vi "Module Loop.vi"(8 "error in (no error)":errorcluster, 11 "System Status Module in":refnum<class "System Status Module.lvclass">) -> (0 "error out":errorcluster, 3 "System Status Module out":refnum<class "System Status Module.lvclass">)   [LabVIEW 2020, in "VolatusGUI.lvlib" / "System Status Module.lvclass"]
uses:
  System Status Module.lvclass
  C:/dev/lv20CE/relink/lv-volatus/Volatus/Module/Module.lvclass
  Client Row.ctl
  Volatus/Module/Module.lvclass/Module.ctl
  Volatus/MessageQ/MessageQ.lvclass/MessageQ.ctl
  System Status Module.lvclass/System Status Module.ctl
  Volatus/Module/Module.lvclass
  Config Updater Identity/Config Updater Identity.lvclass
  C:/dev/lv20CE/relink/lv-volatus/Volatus/Identity/Identity.lvclass
  <vilib>/Utility/error.llb/Error Cluster From Error Code.vi
  Volatus/MessageQ/MessageQ.lvclass
  GUI Helper/GUI Helper.lvclass
  Volatus/VolatusAPI/VolatusAPI.lvclass
  Volatus/Volatus.lvlib
panel:
  in  "Reload Config":bool
  in  "Manage Config":bool
  in  "Clients":T1[](array[typedef])
  # "Node"
  # "Alias"
  # "IP"
  # "App Ver"
  # "Cfg Ver"
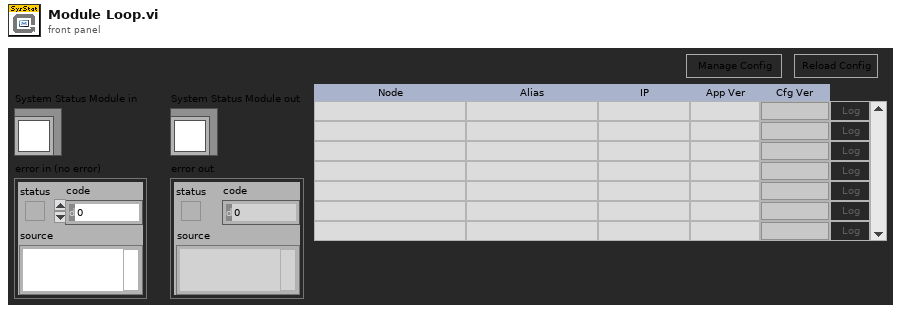
[diagram p1: front panel]
types:
  T1 = typedef "VolatusGUI.lvlib/System Status Module.lvclass/Client Row.ctl" = cluster{"Node":string, "Alias":string, "IP":string, "App Version":string, "Cfg Version":string, "Debug Log":bool, "Cfg Color":u32}
  T2 = enum32{"Invalid", "Standard", "Closed", "Hidden", "Minimized", "Maximized"}
  T3 = cluster{"Node":bool, "Alias":bool, "IP":bool, "App Version":bool, "Cfg Version":bool, "Debug Log":bool, "Cfg Color":bool}[]
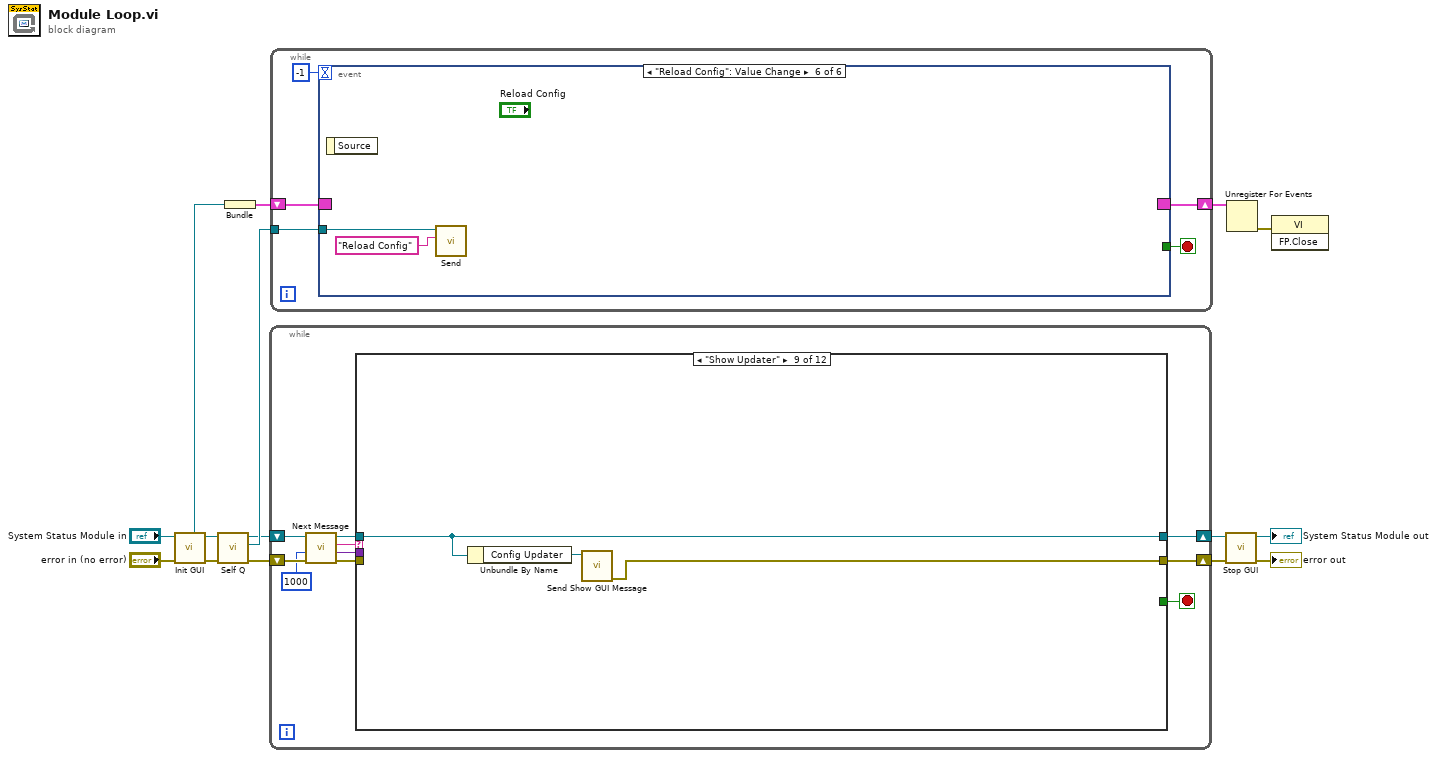
[diagram p0: block diagram]
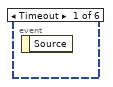
[diagram p2: hidden frame]
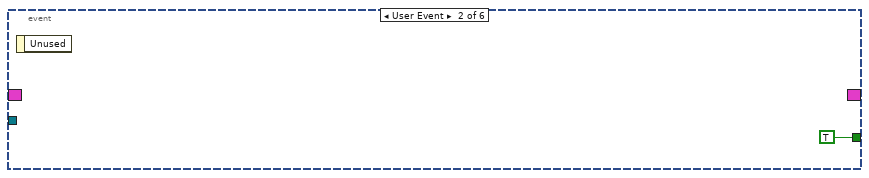
[diagram p3: hidden frame]
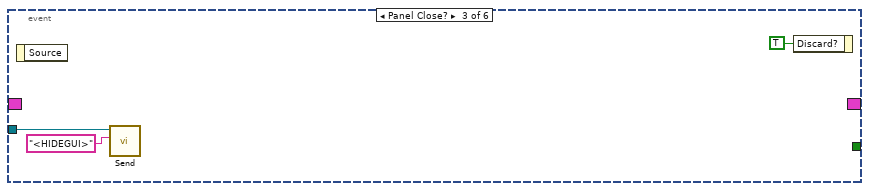
[diagram p4: hidden frame]
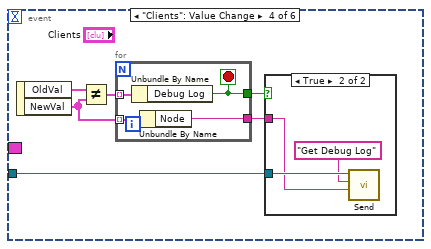
[diagram p5: hidden frame]
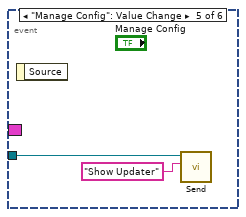
[diagram p7: hidden frame]
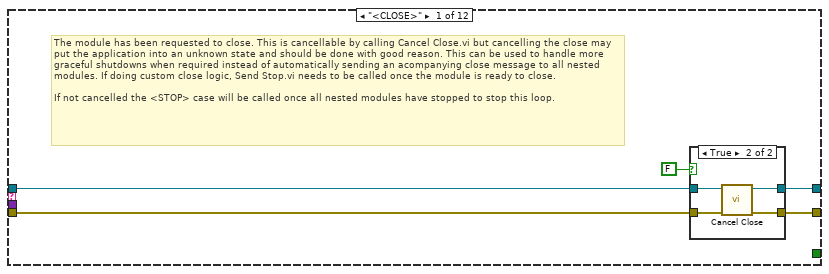
[diagram p8: hidden frame]
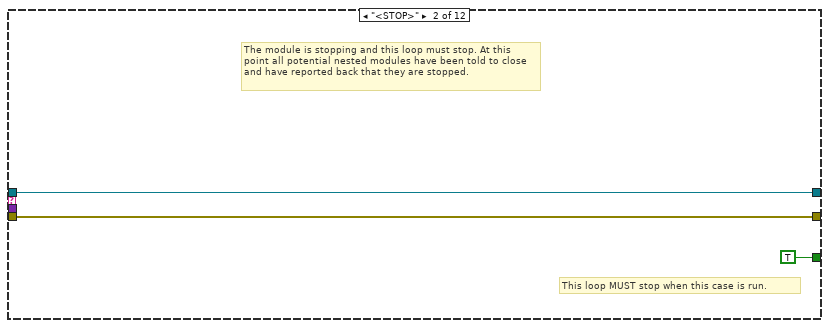
[diagram p10: hidden frame]
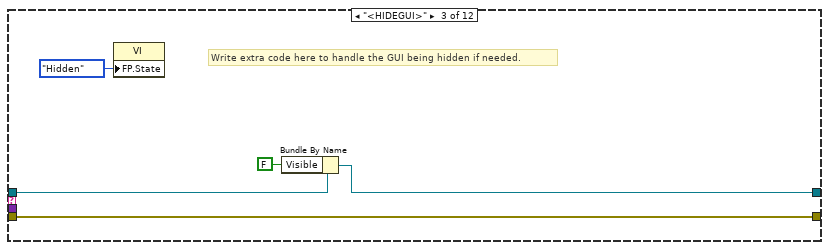
[diagram p11: hidden frame]
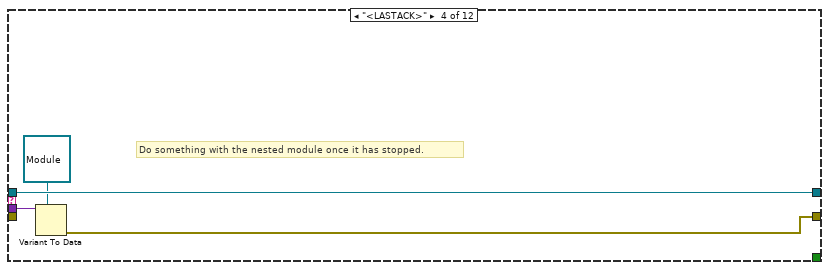
[diagram p12: hidden frame]
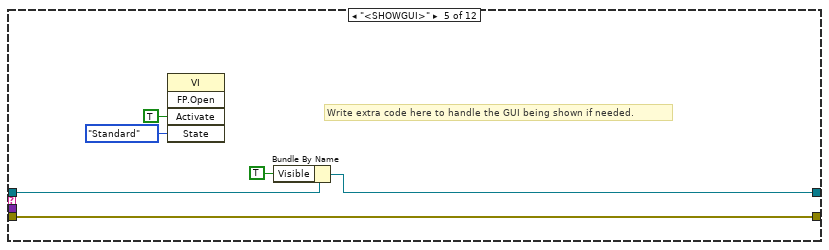
[diagram p13: hidden frame]
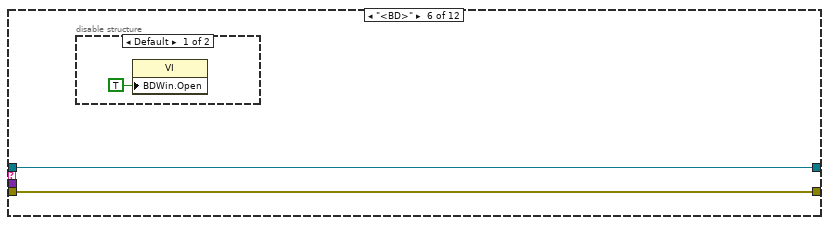
[diagram p14: hidden frame]
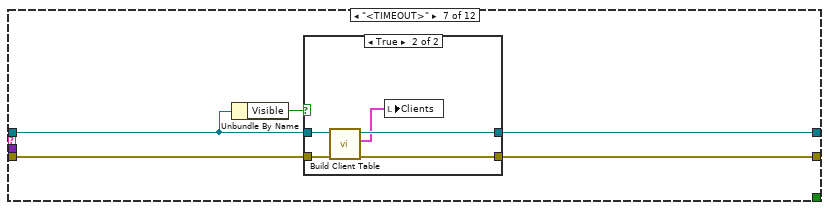
[diagram p16: hidden frame]
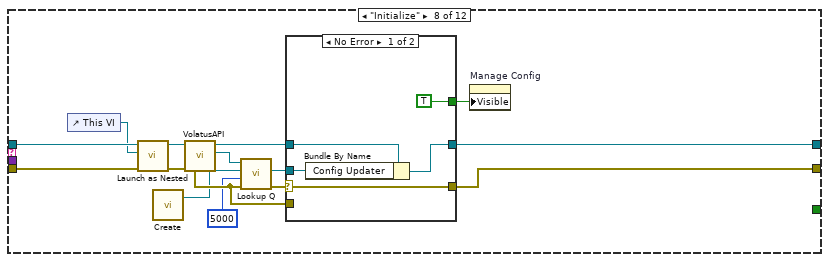
[diagram p18: hidden frame]
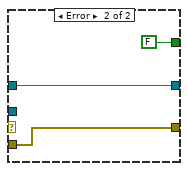
[diagram p19: hidden frame]
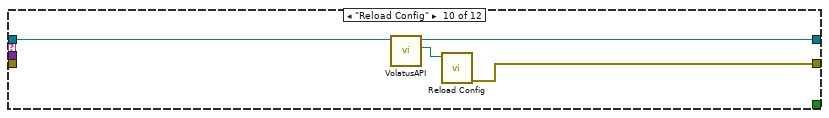
[diagram p20: hidden frame]
diagram:
  n1 = call "Init GUI.vi"("Module in"="System Status Module in") -> ("Module out"=w7:refnum<class "System Status Module.lvclass">, "Event Reg"=w12:refnum<event-registration>)  [unwired: 9 in]
  n2 = call "Self Q.vi"("Module in"=w7) -> ("Self Q"=w6:refnum<class "MessageQ.lvclass">, "Module out"=w5:refnum<class "System Status Module.lvclass">)  [unwired: 9 in]
  n3 = Bundle("Event Reg"=w12) -> (w8:cluster{"Event Reg":refnum<event-registration>})  [unwired: 1 in]
  n4 = while {
    shift-right: [w18] -> w10
    shift-left: w5 -> [w23]
    shift-right: [w17] -> w11
    shift-left: "error in (no error)" -> [w22]
    stop <- w16 stop-if-true
    n5 = call "Next Message.vi"("error in (no error)"=w22, "Timeout ms (-1)"=1000, "Module in"=w23) -> ("error out"=w21:errorcluster, "Data"=w15:variant, "ID"=w20:string, "Module out"=w19:refnum<class "System Status Module.lvclass">)  [unwired: 5 in]
    n6 = case shown="\"Show Updater\"" w20 {
      tunnel: w21 -> [w26 w36 w41 _ w51 w53 w60 w80 _ _ _ w107]
      tunnel: w19 -> [w27 w37 w42 w46 w52 w54 w57 w79 w92 w96 w103 w105]
      tunnel: [w25 w37 w39 w46 w48 w54 w58 w72 w92 w95 w100 w104] -> w18
      tunnel: [w24 w36 w41 w43 w51 w53 w59 w69 w90 w93 w97 w106] -> w17
      tunnel: [_ TRUE _ _ _ _ _ _ _ _ _ _] -> w16
      tunnel: w15 -> [_ _ _ w45 _ _ _ _ _ _ w102 _]
      frame "<CLOSE>" {
        # "The module has been requested to close. This is cancellable by calling Cancel Close.vi but cancelling the close may put the application into an unknown state and should be done with good reason. This can be used to handle more graceful shutdowns when required instead of automatically sending an acompanying close message to all nested modules. If doing custom close logic, Send Stop.vi needs to be called once the module is ready to close.\n\nIf not cancelled the <STOP> case will be called once all nested modules have stopped to stop this loop."
        n7 = case shown="True" FALSE {
          tunnel: w26 -> [w29 w34]
          tunnel: [w29 w33] -> w24
          tunnel: w27 -> [w30 w32]
          tunnel: [w30 w31] -> w25
          frame False {
          }
          frame True {
            n8 = call "Cancel Close.vi"("error in (no error)"=w34, "Module in"=w32) -> ("error out"=w33:errorcluster, "Module out"=w31:refnum<class "System Status Module.lvclass">)  [unwired: 8 in]
          }
        }
      }
      frame "<STOP>" {
        # "This loop MUST stop when this case is run."
        # "The module is stopping and this loop must stop. At this point all potential nested modules have been told to close and have reported back that they are stopped."
      }
      frame "<HIDEGUI>" {
        # "Write extra code here to handle the GUI being hidden if needed."
        n9 = property class="VI"("FP.State"=T2."Hidden" ("Front Panel Window:State")) -> ()  [unwired: 2 in, 2 out]
        n10 = Bundle By Name(cluster=w42, "Visible"=FALSE) -> (w39:refnum<class "System Status Module.lvclass">)
      }
      frame "<LASTACK>" {
        # "Do something with the nested module once it has stopped."
        n11 = Variant To Data(type=refnum<class "Module.lvclass"> refnum ("Volatus:Module"), Variant=w45) -> (error out=w43:errorcluster)  [unwired: 1 in, 1 out]
      }
      frame "<SHOWGUI>" {
        # "Write extra code here to handle the GUI being shown if needed."
        n12 = invoke class="VI" method="FP.Open"("Activate"=TRUE ("Activate?"), "State"=T2."Standard") -> ()  [unwired: 3 in, 5 out]
        n13 = Bundle By Name(cluster=w52, "Visible"=TRUE) -> (w48:refnum<class "System Status Module.lvclass">)
      }
      frame "<BD>" {
        n14 = disable-structure shown="Default" {
          frame condition #0 (active) {
            n15 = property class="VI"("BDWin.Open"=TRUE ("Block Diagram Window:Open")) -> ()  [unwired: 2 in, 2 out]
          }
          frame condition #1 {
          }
        }
      }
      frame "<TIMEOUT>" {
        n16 = Unbundle By Name(w57) -> ("Visible"=w56:bool)
        n17 = case shown="True" w56 {
          tunnel: w60 -> [w61 w67]
          tunnel: [w61 w66] -> w59
          tunnel: [w62 w65] -> w58
          tunnel: w57 -> [w62 w64]
          frame False {
          }
          frame True {
            n18 = call "Build Client Table.vi"("error in (no error)"=w67, "System Status Module in"=w64) -> ("error out"=w66:errorcluster, "Clients"=w63:T1[], "System Status Module out"=w65:refnum<class "System Status Module.lvclass">)  [unwired: 7 in]
            n19 = local write "Clients"(w63) -> ()
          }
        }
      }
      frame "Initialize" {
        n20 = control-ref of="This VI"() -> (w77:refnum<vi>)
        n21 = call "Launch as Nested.vi"("error in (no error)"=w80, "GUI"=w77, "Parent in"=w79) -> ("error out"=w81:errorcluster, "Parent"=w78:refnum<class "System Status Module.lvclass">)  [unwired: 6 in, 1 out]
        n22 = call "Create.vi"() -> ("Config Updater Identity"=w73:refnum<class "Config Updater Identity.lvclass">)  [unwired: 7 in]
        n23 = call "VolatusAPI.vi"("Module in"=w78) -> ("VolatusAPI"=w75:refnum<class "VolatusAPI.lvclass">, "Module out"=w76:refnum<class "System Status Module.lvclass">)  [unwired: 9 in]
        n24 = call "Lookup Q.vi"("error in (no error)"=w81, "Timeout ms (0)"=5000, "Identity"=w73, "VolatusAPI in"=w75) -> ("error out"=w70:errorcluster, "MessageQ"=w71:refnum<class "MessageQ.lvclass">)  [unwired: 5 in, 1 out]
        n25 = case shown="No Error" w70 {
          selector: w70 -> [w83 _]
          tunnel: w76 -> [w86 w88]
          tunnel: [w85 w88] -> w72
          tunnel: w71 -> [w84 _]
          tunnel: [w83 w89] -> w69
          tunnel: w81 -> [_ w89]
          tunnel: [TRUE FALSE] -> w68
          frame No Error {
            n26 = Bundle By Name(cluster=w86, "Config Updater"=w84) -> (w85:refnum<class "System Status Module.lvclass">)
          }
          frame Error {
          }
        }
        n27 = property on="Manage Config" class="Bool"("Visible"=w68) -> ()  [unwired: 2 in, 2 out]
      }
      frame "Show Updater" {
        n28 = Unbundle By Name(w92) -> ("Config Updater"=w91:refnum<class "MessageQ.lvclass">)
        n29 = call "Send Show GUI Message.vi"("MessageQ"=w91) -> ("error out"=w90:errorcluster)  [unwired: 10 in]
      }
      frame "Reload Config" {
        n30 = call "VolatusAPI.vi"("Module in"=w96) -> ("VolatusAPI"=w94:refnum<class "VolatusAPI.lvclass">, "Module out"=w95:refnum<class "System Status Module.lvclass">)  [unwired: 9 in]
        n31 = call "Reload Config.vi"("VolatusAPI in"=w94) -> ("error out"=w93:errorcluster)  [unwired: 9 in, 1 out]
      }
      frame "Get Debug Log" {
        n32 = Variant To Data(type="", Variant=w102) -> (data=w99:string, error out=w98:errorcluster)  [unwired: 1 in]
        n33 = call "Get Debug Log.vi"("error in (no error)"=w98, "Node"=w99, "System Status Module in"=w103) -> ("error out"=w97:errorcluster, "System Status Module out"=w100:refnum<class "System Status Module.lvclass">)  [unwired: 7 in]
      }
      frame Default {
        n34 = call "Report Unhandled Message ID.vi"("error in (no error)"=w107, "Module in"=w105) -> ("error out"=w106:errorcluster, "Module out"=w104:refnum<class "System Status Module.lvclass">)  [unwired: 8 in]
      }
    }
  }
  n35 = while {
    tunnel: w6 -> [w112]
    shift-right: [w110] -> w9
    shift-left: w8 -> [w111]
    stop <- w109 stop-if-true
    n36 = event shown="[5] \"Reload Config\": Value Change" {
      selector: w111 -> [_ _ _ _ _ _]
      dyn-events: [_ _ _ _ _ _] -> w110
      timeout: -1 -> [_ _ _ _ _ _]
      tunnel: w112 -> [_ _ w115 w117 w131 w133]
      tunnel: [_ TRUE _ _ _ _] -> w109
      event Timeout {
        n37 = event-data() -> ()  [unwired: 1 in, 1 out]
      }
      event User Event {
        n38 = event-data() -> ()  [unwired: 1 in, 1 out]
      }
      event Panel Close? {
        n39 = event-data() -> ()  [unwired: 1 in, 1 out]
        n40 = call "Send.vi"("ID"="<HIDEGUI>", "MessageQ in"=w115) -> ()  [unwired: 8 in, 2 out]
        n41 = event-data("Discard?"=TRUE) -> ()  [unwired: 1 in, 1 out]
      }
      event "Clients": Value Change {
        n42 = event-data() -> ("OldVal"=w122:T1[], "NewVal"=w120:T1[])  [unwired: 1 in]
        n43 = Not Equal?(x=w122, y=w120) -> (x != y?=w121:T3)
        n44 = for {
          tunnel: w121 -> [w129] mode=indexing
          tunnel: w120 -> [w128] mode=indexing
          tunnel: [w127] -> w118
          tunnel: [w126] -> w119
          stop <- w126 stop-if-true
          n45 = Unbundle By Name(w129) -> ("Debug Log"=w126:bool)
          n46 = Unbundle By Name(w128) -> ("Node"=w127:string)
        }
        n47 = case shown="True" w119 {
          tunnel: w118 -> [_ w123]
          tunnel: w117 -> [_ w125]
          frame False {
          }
          frame True {
            n48 = call "Send.vi"("Data"=w123, "ID"="Get Debug Log", "MessageQ in"=w125) -> ()  [unwired: 7 in, 2 out]
          }
        }
      }
      event "Manage Config": Value Change {
        n49 = event-data() -> ()  [unwired: 1 in, 1 out]
        n50 = call "Send.vi"("ID"="Show Updater", "MessageQ in"=w131) -> ()  [unwired: 8 in, 2 out]
      }
      event "Reload Config": Value Change {
        n51 = event-data() -> ()  [unwired: 1 in, 1 out]
        n52 = call "Send.vi"("ID"="Reload Config", "MessageQ in"=w133) -> ()  [unwired: 8 in, 2 out]
      }
    }
  }
  n53 = call "Stop GUI.vi"("error in (no error)"=w11, "Module in"=w10) -> ("error out"=→"error out":errorcluster, "Module out"=→"System Status Module out":refnum<class "System Status Module.lvclass">)  [unwired: 8 in]
  n54 = Unregister For Events(event registration refnum=w9) -> (error out=w13:errorcluster)  [unwired: 1 in]
  n55 = invoke class="VI" method="FP.Close"(error in=w13) -> ()  [unwired: 2 in, 3 out]
